vi "Get PDO Mapping.vi"(8 "error in":errorcluster, 11 "Object Entry in":refnum<class "Object Entry.lvclass">) -> (0 "error out":errorcluster, 2 "PDO Mapping":bool, 3 "Object Entry out":refnum<class "Object Entry.lvclass">)   [LabVIEW 2020, in "CANopen.lvlib" / "Object Entry.lvclass"]
uses:
  Object Entry.lvclass
  Object Entry.lvclass/Object Entry.ctl
  Sub Object/Sub Object.lvclass
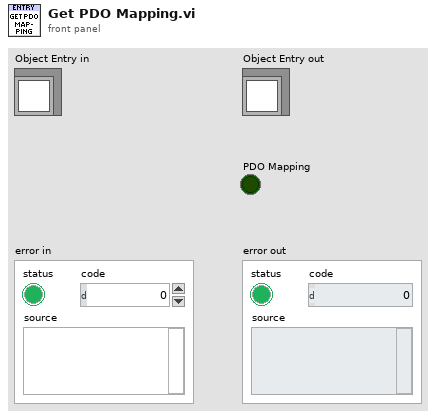
[diagram p1: front panel]
types:
  T1 = typedef "CANopen.lvlib/Object Type.ctl" = u8
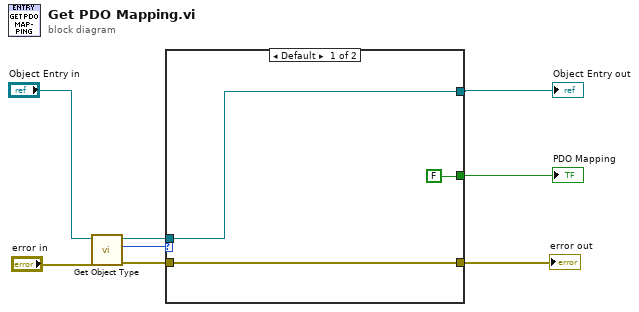
[diagram p0: block diagram]
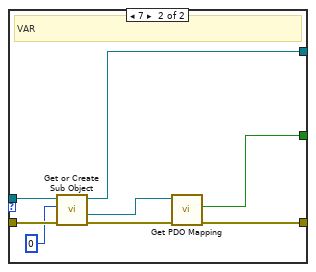
[diagram p2: hidden frame]
diagram:
  n1 = call "Get Object Type.vi"("error in"="error in", "Object Entry in"="Object Entry in") -> ("error out"=w6:errorcluster, "Object Type"=w7:T1, "Object Entry out"=w8:refnum<class "Object Entry.lvclass">)  [unwired: 7 in]
  n2 = case shown="Default" w7 {
    tunnel: w8 -> [w10 w17]
    tunnel: [w10 w16] -> w1
    tunnel: w6 -> [w11 w19]
    tunnel: [w11 w14] -> w2
    tunnel: [FALSE ("PDO Mapping") w12] -> w3
    frame Default {
    }
    frame 7 {
      # "VAR"
      n3 = call "Get or Create Sub Object.vi"("error in"=w19, "Sub Index"=u8 0, "Obj Entry in"=w17) -> ("error out"=w18:errorcluster, "Sub Object"=w13:refnum<class "Sub Object.lvclass">, "Obj Entry out"=w16:refnum<class "Object Entry.lvclass">)  [unwired: 6 in]
      n4 = call "Get PDO Mapping.vi"("error in"=w18, "Sub Object in"=w13) -> ("error out"=w14:errorcluster, "PDO Mapping"=w12:bool)  [unwired: 7 in, 1 out]
    }
  }
  "error out" <- w2
  "Object Entry out" <- w1
  "PDO Mapping" <- w3
